vi "New SN3218.vi"(8 "error in (no error)":errorcluster, 11 "I2C":refnum<class "LINX I2C.lvclass">) -> (0 "error out":errorcluster, 3 "LINX-SN3218 out":refnum<class "LINX-SN3218.lvclass">)   [LabVIEW 2020, in "LINX-SN3218.lvclass"]
doc: "Creates a new instance of the SN3218 device from the configured I2C channel."
uses:
  LINX-SN3218.lvclass
  LINX I2C/LINX I2C.lvclass
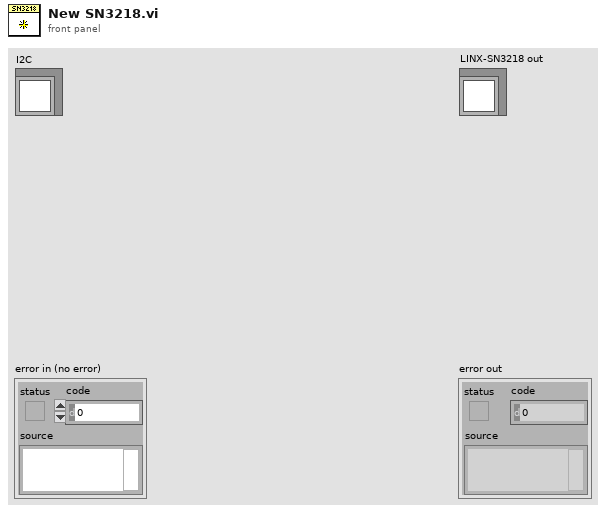
[diagram p1: front panel]
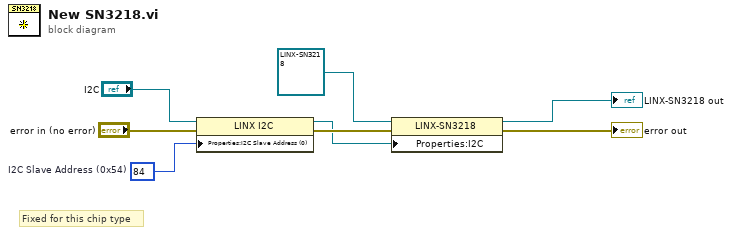
[diagram p0: block diagram]
diagram:
  w6 = u8 84  # I2C Slave Address (0x54)
  # "Fixed for this chip type"
  n1 = property class="LINX I2C"(reference="I2C", error in="error in (no error)", "Properties:I2C Slave Address (0)"=w6) -> (reference out=w5:refnum<class "LINX I2C.lvclass">, error out=w8:errorcluster)
  n2 = property class="LINX-SN3218"(reference=refnum<class "LINX-SN3218.lvclass"> refnum ("LINX-SN3218 in"), error in=w8, "Properties:I2C"=w5) -> (reference out=→"LINX-SN3218 out":refnum<class "LINX-SN3218.lvclass">, error out=→"error out":errorcluster)
